vi "Apply_Source.vi"(8 "error in (no error)":errorcluster, 9 "source":refnum<class "IB_Source.lvclass">, 10 "address":string, 11 "Installer in":refnum<class "Installer.lvclass">) -> (0 "error out":errorcluster, 2 "address out":string, 3 "Installer out":refnum<class "Installer.lvclass">)   [LabVIEW 2020, in "Installer.lvclass"]
uses:
  <vilib>/AppBuilder/IB_Classes/Installer/Installer.lvclass
  <vilib>/AppBuilder/IB_Classes/Installer/Installer.lvclass/Installer.ctl
  <vilib>/AppBuilder/IB_Classes/Source/IB_Source.lvclass
  <vilib>/AppBuilder/IB_Classes/Source/Container/IB_Source_Container.lvclass
  <vilib>/AppBuilder/IB_Classes/Source/File/CtrFile/IB_CtrFile.lvclass
  e:/builds/penguin/labview/branches/2020/dev/dist/vi.lib/AppBuilder/IB_Classes/Source/File/IB_Source_File.lvclass
  e:/builds/penguin/labview/branches/2020/dev/dist/vi.lib/AppBuilder/IB_Classes/Source/IB_Source.lvclass
  e:/builds/penguin/labview/branches/2020/dev/dist/vi.lib/AppBuilder/IB_Classes/Source/File/CtrFile/IB_CtrFile.lvclass
  e:/builds/penguin/labview/branches/2020/dev/dist/vi.lib/AppBuilder/IB_Classes/Source/Container/IB_Source_Container.lvclass
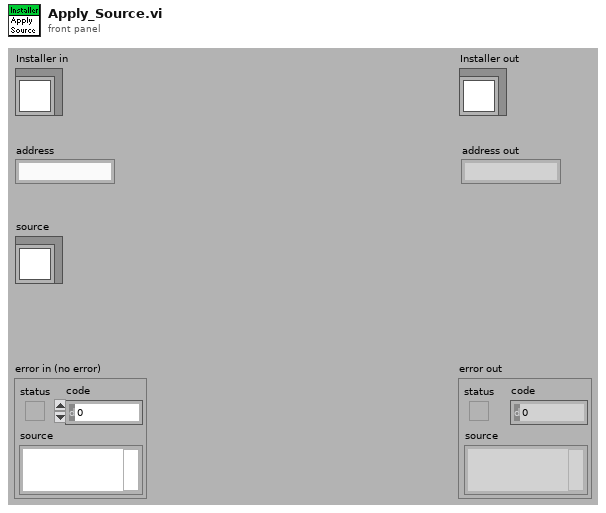
[diagram p1: front panel]
types:
  T1 = typedef "IB_Source.ctl" = cluster{"name":string, "sourceTag":string, "destTag":string, "path":path, "eng_installPath":string, "UI_inBuild?":bool, "str ref?":bool}
  T2 = typedef "IB_Source_Container.ctl" = cluster{"files":refnum<class "IB_CtrFile.lvclass">[], "previewed?":bool, "preview error?":bool}
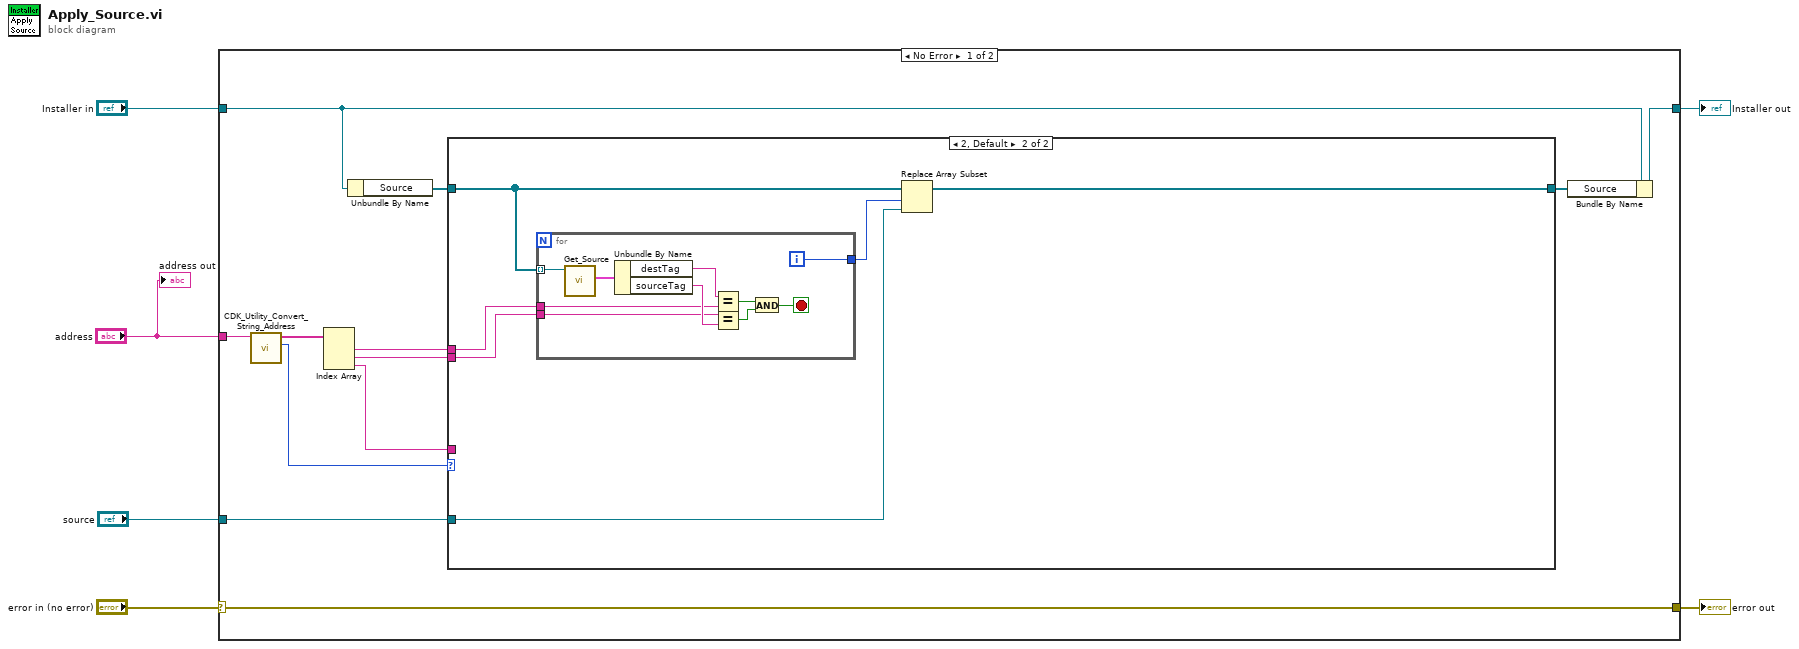
[diagram p0: block diagram]
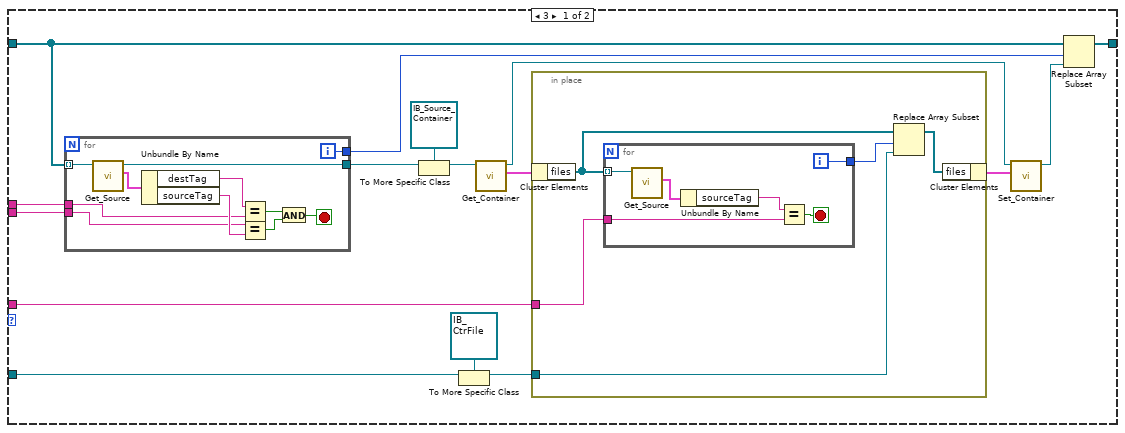
[diagram p2: hidden frame]
diagram:
  n1 = case shown="No Error" "error in (no error)" {
    selector: "error in (no error)" -> [w18 w74]
    tunnel: [w18 w74] -> w5
    tunnel: [w16 w73] -> w3
    tunnel: "Installer in" -> [w17 w73]
    tunnel: "address" -> [w10 _]
    tunnel: "source" -> [w14 _]
    frame No Error {
      n2 = call <resource>:"CDK_Utility_Convert_String_Address.vi"("address"=w10) -> ("address size"=w9:i32, "address parts"=w8:string[])  [unwired: 9 out]
      n3 = Index Array(array=w8) -> (element #1=w7:string, element #2=w11:string, element #3=w13:string)  [unwired: 3 in]
      n4 = Unbundle By Name(w17) -> ("Source"=w12:refnum<class "IB_Source.lvclass">[])
      n5 = case shown="2, Default" w9 {
        tunnel: [w20 w62] -> w15
        tunnel: w14 -> [w28 w61]
        tunnel: w13 -> [w30 _]
        tunnel: w12 -> [w21 w59]
        tunnel: w11 -> [w31 w58]
        tunnel: w7 -> [w19 w57]
        frame 3 {
          n6 = for {
            tunnel: w21 -> [w56] mode=indexing
            tunnel: w31 -> [w46]
            tunnel: [w55] -> w32
            tunnel: [w54] -> w22
            tunnel: w19 -> [w47]
            i -> [w54]
            stop <- w48 stop-if-true
            n7 = call <vilib>:"Get_Source.vi"("IB_Source in"=w56) -> ("data"=w49:T1, "IB_Source out"=w55:refnum<class "IB_Source.lvclass">)  [unwired: 1 in, 8 out]
            n8 = Unbundle By Name(w49) -> ("destTag"=w50:string, "sourceTag"=w51:string)
            n9 = Equal?(x=w50, y=w47) -> (x = y?=w52:bool)
            n10 = Equal?(x=w46, y=w51) -> (x = y?=w53:bool)
            n11 = And(x=w52, y=w53) -> (x .and. y?=w48:bool)
          }
          n12 = To More Specific Class(target class=refnum<class "IB_Source_Container.lvclass"> refnum ("IB_Source_Container.lvclass"), reference=w32) -> (specific class reference=w34:refnum<class "IB_Source_Container.lvclass">)  [unwired: 1 in, 1 out]
          n13 = To More Specific Class(target class=refnum<class "IB_CtrFile.lvclass"> refnum ("IB_CtrFile.lvclass"), reference=w28) -> (specific class reference=w27:refnum<class "IB_CtrFile.lvclass">)  [unwired: 1 in, 1 out]
          n14 = call <vilib>:"Get_Container.vi"("IB_Source_Container in"=w34) -> ("data"=w26:T2, "IB_Source_Container out"=w25:refnum<class "IB_Source_Container.lvclass">)  [unwired: 1 in, 8 out]
          n15 = in-place {
            in-place-border: w30 -> [w39]
            in-place-border: w27 -> [w37]
            n16 = in-place-cluster #1(w26) -> ("files"=w36:refnum<class "IB_CtrFile.lvclass">[])
            n17 = for {
              tunnel: w36 -> [w45] mode=indexing
              tunnel: w39 -> [w43]
              tunnel: [w40] -> w38
              i -> [w40]
              stop <- w41 stop-if-true
              n18 = call <vilib>:"Get_Source.vi"("IB_Source in"=w45) -> ("data"=w42:T1)  [unwired: 1 in, 9 out]
              n19 = Unbundle By Name(w42) -> ("sourceTag"=w44:string)
              n20 = Equal?(x=w44, y=w43) -> (x = y?=w41:bool)
            }
            n21 = Replace Array Subset(array=w36, new element=w37, index=w38) -> (w35:refnum<class "IB_CtrFile.lvclass">[])
            n22 = in-place-cluster #1("files"=w35) -> (w24:T2)
          }
          n23 = call <vilib>:"Set_Container.vi"("data"=w24, "IB_Source_Container in"=w25) -> ("IB_Source_Container out"=w23:refnum<class "IB_Source_Container.lvclass">)  [unwired: 1 in, 8 out]
          n24 = Replace Array Subset(array=w21, new element=w23, index=w22) -> (w20:refnum<class "IB_Source.lvclass">[])
        }
        frame 2, Default {
          n25 = for {
            tunnel: w59 -> [w72] mode=indexing
            tunnel: w58 -> [w65]
            tunnel: [w71] -> w60
            tunnel: w57 -> [w64]
            i -> [w71]
            stop <- w63 stop-if-true
            n26 = call <vilib>:"Get_Source.vi"("IB_Source in"=w72) -> ("data"=w66:T1)  [unwired: 1 in, 9 out]
            n27 = Unbundle By Name(w66) -> ("destTag"=w67:string, "sourceTag"=w68:string)
            n28 = Equal?(x=w67, y=w64) -> (x = y?=w69:bool)
            n29 = Equal?(x=w65, y=w68) -> (x = y?=w70:bool)
            n30 = And(x=w69, y=w70) -> (x .and. y?=w63:bool)
          }
          n31 = Replace Array Subset(array=w59, new element=w61, index=w60) -> (w62:refnum<class "IB_Source.lvclass">[])
        }
      }
      n32 = Bundle By Name(cluster=w17, "Source"=w15) -> (w16:refnum<class "Installer.lvclass">)
    }
    frame Error {
    }
  }
  "error out" <- w5
  "Installer out" <- w3
  "address out" <- "address"
